vi "Cleanup.vi"(8 "error in (no error)":errorcluster, 11 "Menu in":refnum<class "MGI_Menu.lvclass">) -> (0 "error out":errorcluster)   [LabVIEW 2016, in "MGI_Menu.lvclass"]
doc: "Destroys the Menu and all MenuItems inside it.\n\nAuthored by Derek E. Trepanier\nsupport@mooregoodideas.com\nwww.mooregoodideas.com\n\nCopyright (c) 2012, Moore Good Ideas, Inc.\n\nAll rights reserved.\n\nRedistribution and use in source and binary forms, with or without modification, are permitted provided that the following conditions are met:\n\n * Redistributions of source code must retain the above copyright notice, this list of conditions and the following disclaimer.\n * Redistributions in binary form must reproduce the above copyright notice, this list of conditions and the following disclaimer in the documentation and/or other materials provided with the distribution.\n * Neither the name of Moore Good Ideas, Inc. nor the names of its contributors may be used to endorse or promote products derived from this software without specific prior written permission.\n\nTHIS SOFTWARE IS PROVIDED BY THE COPYRIGHT HOLDERS AND CONTRIBUTORS \"AS IS\" AND ANY EXPRESS OR IMPLIED WARRANTIES, INCLUDING, BUT NOT LIMITED TO, THE IMPLIED WARRANTIES OF MERCHANTABILITY AND FITNESS FOR A PARTICULAR PURPOSE ARE DISCLAIMED. IN NO EVENT SHALL THE COPYRIGHT OWNER OR CONTRIBUTORS BE LIABLE FOR ANY DIRECT, INDIRECT, INCIDENTAL, SPECIAL, EXEMPLARY, OR CONSEQUENTIAL DAMAGES (INCLUDING, BUT NOT LIMITED TO, PROCUREMENT OF SUBSTITUTE GOODS OR SERVICES; LOSS OF USE, DATA, OR PROFITS; OR BUSINESS INTERRUPTION) HOWEVER CAUSED AND ON ANY THEORY OF LIABILITY, WHETHER IN CONTRACT, STRICT LIABILITY, OR TORT (INCLUDING NEGLIGENCE OR OTHERWISE) ARISING IN ANY WAY OUT OF THE USE OF THIS SOFTWARE, EVEN IF ADVISED OF THE POSSIBILITY OF SUCH DAMAGE."
uses:
  <userlib>/_MGI/Menu Building/MenuTypes/MGI_Menu.lvclass
  <userlib>/_MGI/Menu Building/MenuTypes/MGI_Menu.lvclass/MGI_Menu.ctl
  <userlib>/_MGI/Menu Building/MenuItem/MGI_MenuItem.lvclass
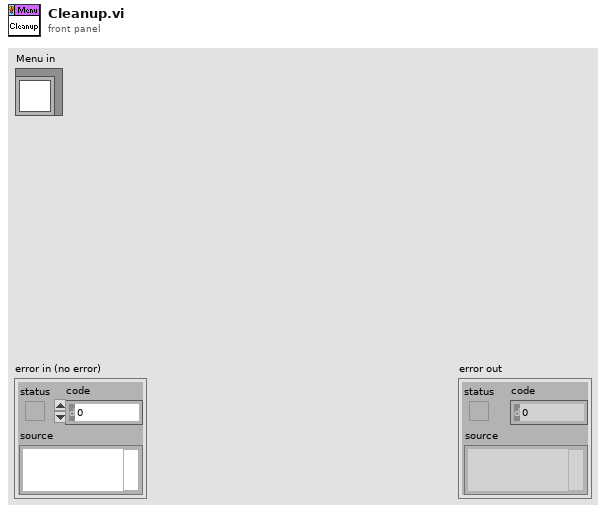
[diagram p1: front panel]
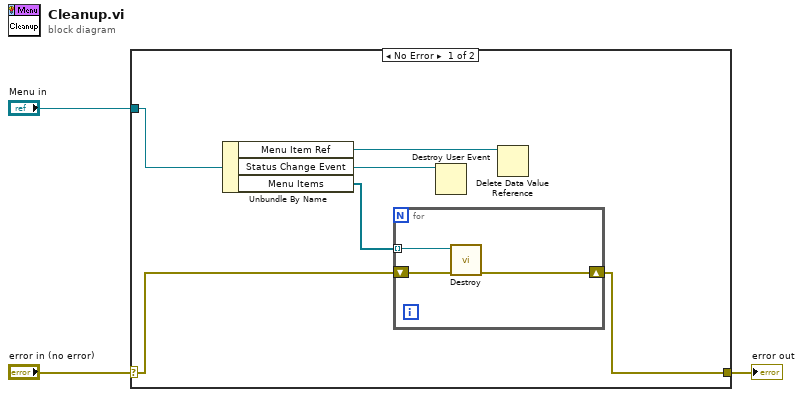
[diagram p0: block diagram]
diagram:
  n1 = case shown="No Error" "error in (no error)" {
    selector: "error in (no error)" -> [w6 w13]
    tunnel: [w5 w13] -> w2
    tunnel: "Menu in" -> [w9 _]
    frame No Error {
      n2 = Unbundle By Name(w9) -> ("Menu Item Ref"=w4:refnum<data-value>, "Status Change Event"=w8:refnum<user-event>, "Menu Items"=w7:refnum<data-value>[])
      n3 = for {
        tunnel: w7 -> [w12] mode=indexing
        shift-right: [w10] -> w5
        shift-left: w6 -> [w11]
        n4 = call <userlib>:"Destroy.vi"("error in (no error)"=w11, "Menu Item ref"=w12) -> ("error out"=w10:errorcluster)  [unwired: 9 in]
      }
      n5 = Destroy User Event(user event=w8) -> ()  [unwired: 1 in, 1 out]
      n6 = Delete Data Value Reference(data value reference=w4) -> ()  [unwired: 1 in, 2 out]
    }
    frame Error {
    }
  }
  "error out" <- w2
